vi "Translate Stamp Calibration.vi"(0 "Known HDI Fiducials Coordinates":T3, 1 "Known Stamp Tool Coordinates":T2, 2 "Known Stamp Offsets":T1) -> (7 "Vec3d String":string, 8 "Orient3d String":string, 9 "brass piece rotation":dbl, 10 "net rotation":dbl)   [LabVIEW 2011]
uses:
  Shared Components/Vec3d Class/Vec3d Class.lvclass
  Shared Components/Orient3d Class/Orient3d Class.lvclass
panel:
  out "Pos Z":dbl
  out "Pos Y":dbl
  out "Pos X":dbl
  out "orient w":dbl
  out "orient z":dbl
  out "orient y":dbl
  out "orient x":dbl
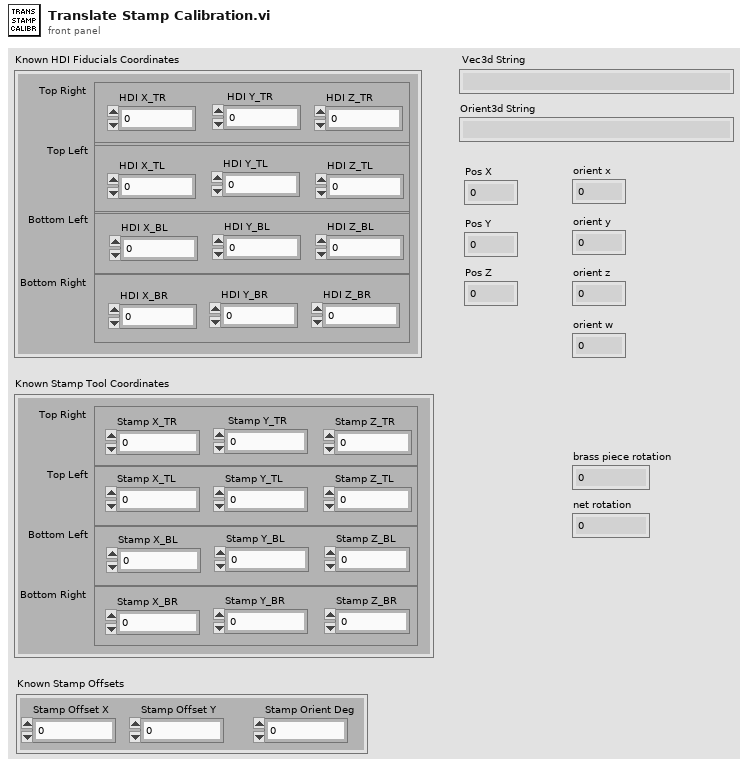
[diagram p1: front panel]
types:
  T1 = cluster{"Stamp Offset X":dbl, "Stamp Offset Y":dbl, "Stamp Orient Deg":dbl}
  T2 = cluster{"Top Right":cluster{"Stamp X_TR":dbl, " Stamp Y_TR":dbl, "Stamp Z_TR":dbl}, "Top Left":cluster{"Stamp X_TL":dbl, "Stamp Y_TL":dbl, "Stamp Z_TL":dbl}, "Bottom Left":cluster{"Stamp X_BL":dbl, "Stamp Y_BL":dbl, "Stamp Z_BL":dbl}, "Bottom Right":cluster{"Stamp X_BR":dbl, "Stamp Y_BR":dbl, "Stamp Z_BR":dbl}}
  T3 = cluster{"Top Right":cluster{"HDI X_TR":dbl, " HDI Y_TR":dbl, "HDI Z_TR":dbl}, "Top Left":cluster{"HDI X_TL":dbl, "HDI Y_TL":dbl, "HDI Z_TL":dbl}, "Bottom Left":cluster{"HDI X_BL":dbl, "HDI Y_BL":dbl, "HDI Z_BL":dbl}, "Bottom Right":cluster{"HDI X_BR":dbl, "HDI Y_BR":dbl, "HDI Z_BR":dbl}}
  T4 = cluster{"Stamp X_TR":dbl, " Stamp Y_TR":dbl, "Stamp Z_TR":dbl}
  T5 = cluster{"Stamp X_TL":dbl, "Stamp Y_TL":dbl, "Stamp Z_TL":dbl}
  T6 = cluster{"Stamp X_BL":dbl, "Stamp Y_BL":dbl, "Stamp Z_BL":dbl}
  T7 = cluster{"Stamp X_BR":dbl, "Stamp Y_BR":dbl, "Stamp Z_BR":dbl}
  T8 = cluster{"HDI X_TR":dbl, " HDI Y_TR":dbl, "HDI Z_TR":dbl}
  T9 = cluster{"HDI X_TL":dbl, "HDI Y_TL":dbl, "HDI Z_TL":dbl}
  T10 = cluster{"HDI X_BL":dbl, "HDI Y_BL":dbl, "HDI Z_BL":dbl}
  T11 = cluster{"HDI X_BR":dbl, "HDI Y_BR":dbl, "HDI Z_BR":dbl}
  T12 = typedef "Position_Orientation.ctl" = cluster{"Center":refnum<class "Vec3d Class.lvclass">, "Orientation":refnum<class "Orient3d Class.lvclass">}
  T13 = typedef "Quaternion.ctl" = cluster{"x":dbl, "y":dbl, "z":dbl, "w":dbl}
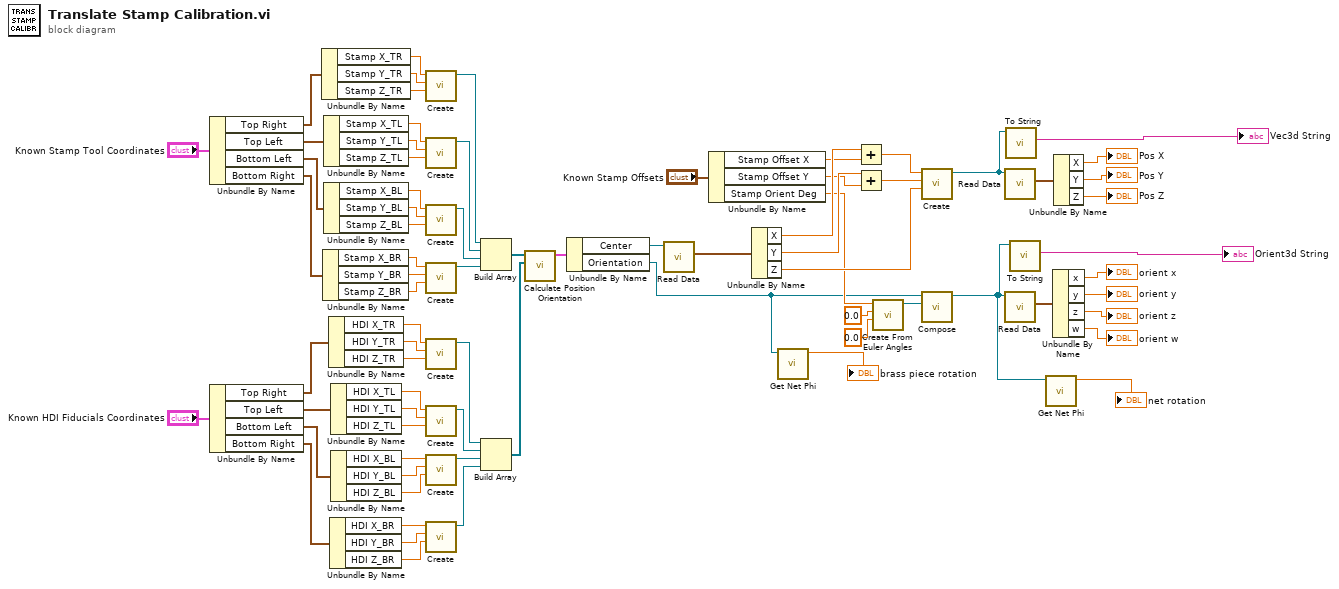
[diagram p0: block diagram]
diagram:
  n1 = Unbundle By Name("Known Stamp Tool Coordinates") -> ("Top Right"=w23:T4, "Top Left"=w22:T5, "Bottom Left"=w21:T6, "Bottom Right"=w20:T7)
  n2 = Unbundle By Name("Known HDI Fiducials Coordinates") -> ("Top Right"=w40:T8, "Top Left"=w36:T9, "Bottom Left"=w29:T10, "Bottom Right"=w25:T11)
  n3 = Unbundle By Name(w23) -> ("Stamp X_TR"=w19:dbl, "Stamp Y_TR"=w18:dbl, "Stamp Z_TR"=w17:dbl)
  n4 = Unbundle By Name(w20) -> ("Stamp X_BR"=w10:dbl, "Stamp Y_BR"=w9:dbl, "Stamp Z_BR"=w8:dbl)
  n5 = Unbundle By Name(w22) -> ("Stamp X_TL"=w16:dbl, "Stamp Y_TL"=w15:dbl, "Stamp Z_TL"=w14:dbl)
  n6 = Unbundle By Name(w21) -> ("Stamp X_BL"=w13:dbl, "Stamp Y_BL"=w12:dbl, "Stamp Z_BL"=w11:dbl)
  n7 = Unbundle By Name(w40) -> ("HDI X_TR"=w39:dbl, "HDI Y_TR"=w38:dbl, "HDI Z_TR"=w37:dbl)
  n8 = Unbundle By Name(w25) -> ("HDI X_BR"=w28:dbl, "HDI Y_BR"=w27:dbl, "HDI Z_BR"=w26:dbl)
  n9 = Unbundle By Name(w36) -> ("HDI X_TL"=w35:dbl, "HDI Y_TL"=w34:dbl, "HDI Z_TL"=w33:dbl)
  n10 = Unbundle By Name(w29) -> ("HDI X_BL"=w32:dbl, "HDI Y_BL"=w31:dbl, "HDI Z_BL"=w30:dbl)
  n11 = call "Create.vi"("Z"=w17, "Y"=w18, "X"=w19) -> ("Vec3d Class out"=w71:refnum<class "Vec3d Class.lvclass">)  [unwired: 7 in, 1 out]
  n12 = call "Create.vi"("Z"=w14, "Y"=w15, "X"=w16) -> ("Vec3d Class out"=w70:refnum<class "Vec3d Class.lvclass">)  [unwired: 7 in, 1 out]
  n13 = call "Create.vi"("Z"=w11, "Y"=w12, "X"=w13) -> ("Vec3d Class out"=w69:refnum<class "Vec3d Class.lvclass">)  [unwired: 7 in, 1 out]
  n14 = call "Create.vi"("Z"=w8, "Y"=w9, "X"=w10) -> ("Vec3d Class out"=w67:refnum<class "Vec3d Class.lvclass">)  [unwired: 7 in, 1 out]
  n15 = call "Create.vi"("Z"=w37, "Y"=w38, "X"=w39) -> ("Vec3d Class out"=w75:refnum<class "Vec3d Class.lvclass">)  [unwired: 7 in, 1 out]
  n16 = call "Create.vi"("Z"=w33, "Y"=w34, "X"=w35) -> ("Vec3d Class out"=w74:refnum<class "Vec3d Class.lvclass">)  [unwired: 7 in, 1 out]
  n17 = call "Create.vi"("Z"=w30, "Y"=w31, "X"=w32) -> ("Vec3d Class out"=w73:refnum<class "Vec3d Class.lvclass">)  [unwired: 7 in, 1 out]
  n18 = call "Create.vi"("Z"=w26, "Y"=w27, "X"=w28) -> ("Vec3d Class out"=w68:refnum<class "Vec3d Class.lvclass">)  [unwired: 7 in, 1 out]
  n19 = Build Array(w71, w70, w69, w67) -> (w66:refnum<class "Vec3d Class.lvclass">[])
  n20 = Build Array(w75, w74, w73, w68) -> (w72:refnum<class "Vec3d Class.lvclass">[])
  n21 = call "Calculate Position Orientation.vi"("Measured Global Positions"=w72, "Known Local Positions"=w66) -> ("PositionOrientation"=w65:T12)  [unwired: 7 in, 2 out]
  n22 = Unbundle By Name(w65) -> ("Center"=w64:refnum<class "Vec3d Class.lvclass">, "Orientation"=w6:refnum<class "Orient3d Class.lvclass">)
  n23 = call-dynamic "Read Data.vi"("Vec3d Class in"=w64) -> ("Data"=w63:cluster{"X":dbl, "Y":dbl, "Z":dbl})  [unwired: 8 in, 2 out]
  n24 = Unbundle By Name("Known Stamp Offsets") -> ("Stamp Offset X"=w45:dbl, "Stamp Offset Y"=w44:dbl, "Stamp Orient Deg"=w43:dbl)
  n25 = Unbundle By Name(w63) -> ("X"=w62:dbl, "Y"=w61:dbl, "Z"=w58:dbl)
  n26 = call "Get Net Phi.vi"("Orient3d"=w6) -> ("phi(deg)"=→"brass piece rotation":dbl)  [unwired: 8 in, 2 out]
  n27 = Add(x=w62, y=w45) -> (x+y=w60:dbl)
  n28 = Add(x=w61, y=w44) -> (x+y=w59:dbl)
  n29 = call "Create From Euler Angles.vi"("phi/roll"=0.0, "theta/pitch"=0.0, "psi/yaw"=w43) -> ("Orient3d out"=w42:refnum<class "Orient3d Class.lvclass">)  [unwired: 7 in, 1 out]
  n30 = call "Create.vi"("Z"=w58, "Y"=w59, "X"=w60) -> ("Vec3d Class out"=w4:refnum<class "Vec3d Class.lvclass">)  [unwired: 7 in, 1 out]
  n31 = call "Compose.vi"("Orient3d 2"=w42, "Orient3d 1"=w6) -> ("Orient3d out"=w2:refnum<class "Orient3d Class.lvclass">)  [unwired: 8 in, 1 out]
  n32 = call-dynamic "Read Data.vi"("Vec3d Class in"=w4) -> ("Data"=w50:cluster{"X":dbl, "Y":dbl, "Z":dbl})  [unwired: 8 in, 2 out]
  n33 = call "Read Data.vi"("Orient3d in"=w2) -> ("Quaternion"=w55:T13)  [unwired: 8 in, 2 out]
  n34 = call "To String.vi"("Vec3d in"=w4) -> ("Vec3d String"=→"Vec3d String":string)  [unwired: 8 in, 2 out]
  n35 = call "To String.vi"("Orient3d in"=w2) -> ("Orient3d String"=→"Orient3d String":string)  [unwired: 8 in, 2 out]
  n36 = call "Get Net Phi.vi"("Orient3d"=w2) -> ("phi(deg)"=→"net rotation":dbl)  [unwired: 8 in, 2 out]
  n37 = Unbundle By Name(w55) -> ("x"=→"orient x":dbl, "y"=→"orient y":dbl, "z"=→"orient z":dbl, "w"=→"orient w":dbl)
  n38 = Unbundle By Name(w50) -> ("X"=→"Pos X":dbl, "Y"=→"Pos Y":dbl, "Z"=→"Pos Z":dbl)
